vi "2023_day04 Expand Winning Cards Recursive (SubVI).vi"(7 "Parent Index":i32, 9 "Winning cards Subet In":i32[](array[numeric]), 10 "Winning cards In":i32[](array[numeric])) -> (2 "# of Winning Cards Out":i32)   [LabVIEW 2021]
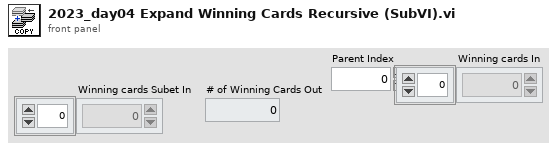
[diagram p1: front panel]
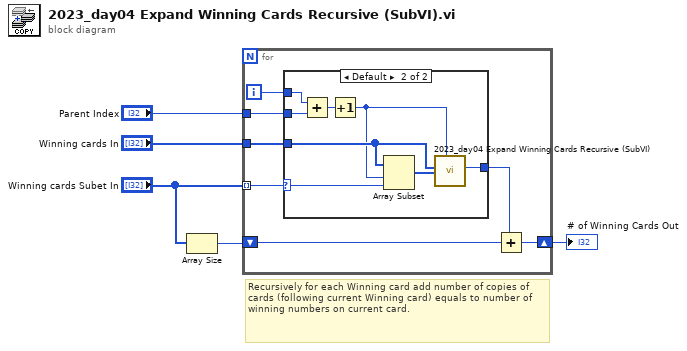
[diagram p0: block diagram]
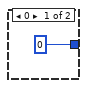
[diagram p2: hidden frame]
diagram:
  # "Recursively for each Winning card add number of copies of cards (following current Winning card) equals to number of winning numbers on current card."
  n1 = Array Size(array="Winning cards Subet In") -> (size(s)=w4:i32)
  n2 = for {
    tunnel: "Winning cards Subet In" -> [w8] mode=indexing
    tunnel: "Winning cards In" -> [w9]
    shift-right: [w12] -> w3
    shift-left: w4 -> [w11]
    tunnel: "Parent Index" -> [w7]
    i -> [w6]
    n3 = case shown="Default" w8 {
      selector: w8 -> [_ w18]
      tunnel: [0 ("# of Winning Cards Out") w21] -> w10
      tunnel: w9 -> [_ w20]
      tunnel: w7 -> [_ w16]
      tunnel: w6 -> [_ w15]
      frame 0 {
      }
      frame Default {
        n4 = Add(x=w15, y=w16) -> (x+y=w17:i32)
        n5 = Increment(x=w17) -> (x+1=w14:i32)
        n6 = Array Subset(array=w20, index=w14, length=w18) -> (w19:i32[])
        n7 = call "2023_day04 Expand Winning Cards Recursive (SubVI).vi"("Parent Index"=w14, "Winning cards Subet In"=w19, "Winning cards In"=w20) -> ("# of Winning Cards Out"=w21:i32)  [unwired: 8 in]
      }
    }
    n8 = Add(x=w10, y=w11) -> (x+y=w12:i32)
  }
  "# of Winning Cards Out" <- w3
